vi "Search Or Add Frame.vi"(10 "Detection Frame in 3":refnum<class "Camera.lvclass">, 11 "Detection Frame in 4":refnum<class "Camera.lvclass">[](array[class])) -> (3 "Detection Frame in 5":refnum<class "Camera.lvclass">[](array[class]))   [LabVIEW 2018]
uses:
  Camera_class/Camera.lvclass
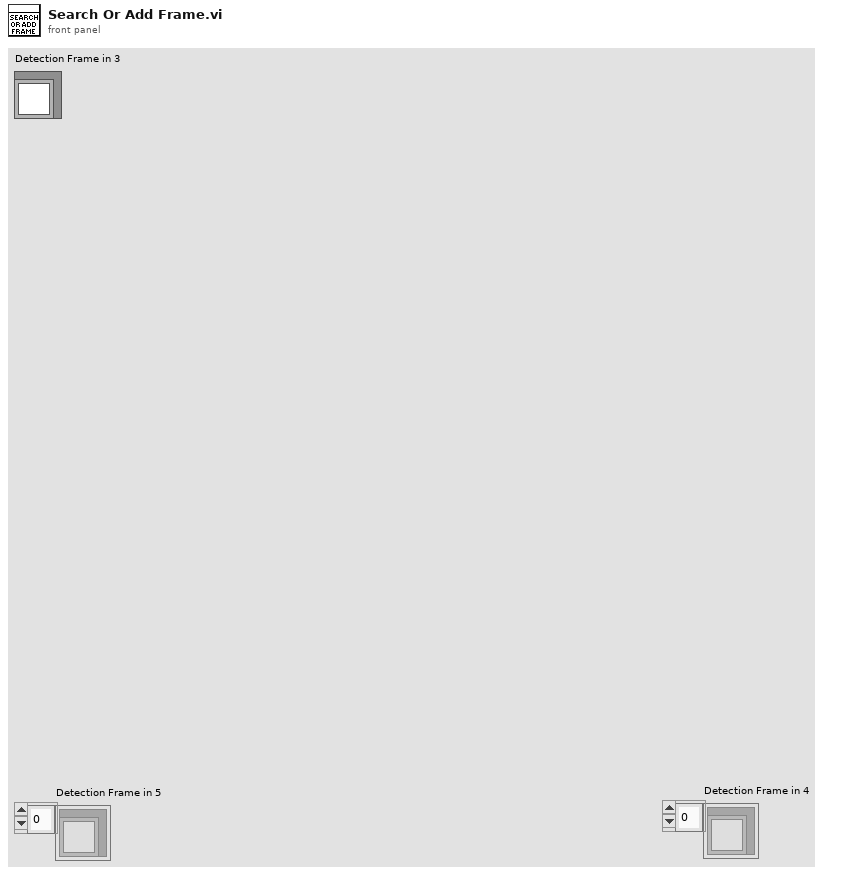
[diagram p1: front panel]
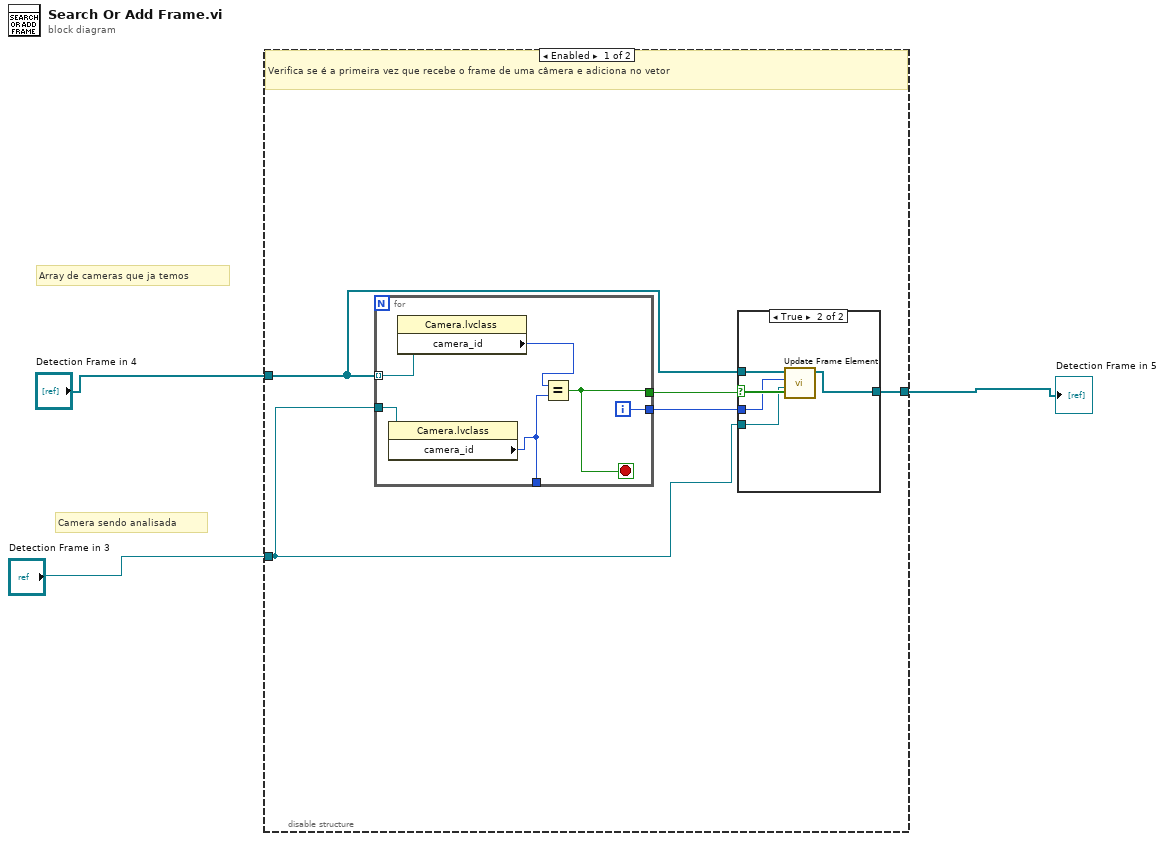
[diagram p0: block diagram]
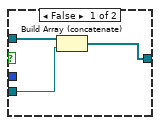
[diagram p2: hidden frame]
diagram:
  # "Camera sendo analisada"
  # "Array de cameras que ja temos"
  n1 = disable-structure "Diagram Disable Structure" shown="Enabled" {
    disable-tunnel: "Detection Frame in 4" -> [w5 _]
    disable-tunnel: "Detection Frame in 3" -> [w4 _]
    disable-tunnel: [w6 _] -> w2
    frame Enabled {
      # "Verifica se é a primeira vez que recebe o frame de uma câmera e adiciona no vetor"
      n2 = for {
        tunnel: w5 -> [w19] mode=indexing
        tunnel: w4 -> [w17]
        tunnel: [w21] -> w8
        tunnel: [w20] -> w7
        tunnel: [w16] -> _
        i -> [w20]
        stop <- w21 stop-if-true
        n3 = property class="Camera.lvclass"(reference=w17) -> ("camera_id"=w16:u32)  [unwired: 1 in, 2 out]
        n4 = property class="Camera.lvclass"(reference=w19) -> ("camera_id"=w18:u32)  [unwired: 1 in, 2 out]
        n5 = Equal?(x=w18, y=w16) -> (x = y?=w21:bool)
      }
      n6 = case shown="True" w8 {
        tunnel: w5 -> [w11 w15]
        tunnel: w4 -> [w10 w13]
        tunnel: [w9 w12] -> w6
        tunnel: w7 -> [_ w14]
        frame False {
          n7 = Build Array (concatenate)(w11, w10) -> (w9:refnum<class "Camera.lvclass">[])
        }
        frame True {
          n8 = call "Update Frame Element.vi"("Detection Frame In in"=w13, "Numeric"=w14, "Detection Frame in 3"=w15) -> ("Detection Frame in out"=w12:refnum<class "Camera.lvclass">[])  [unwired: 8 in]
        }
      }
    }
    frame Disabled {
    }
  }
  "Detection Frame in 5" <- w2
